vi "solar_type Set Items (Variants).vi"(4 "Include Cluster Prefix? (F)":bool, 6 "Prefix":string, 8 "error in (no error)":errorcluster, 9 "Keep Attributes? (F)":bool, 10 "Items":T1[](array[typedef]), 11 "Variant in":variant) -> (0 "error out":errorcluster, 3 "Variant out":variant)   [LabVIEW 2018]
doc: "This sets the Items into the Variant data."
uses:
  solar_type Item Type.ctl
  solar_type Item.ctl
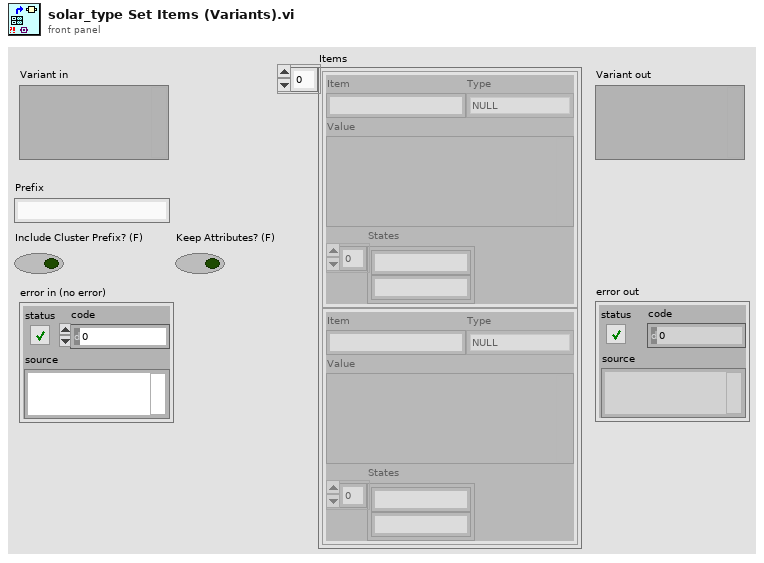
[diagram p1: front panel]
types:
  T1 = typedef "solar_type Item.ctl" = cluster{"Item":string, "Type":T2, "Value":variant, "States":string[]}
  T2 = typedef "solar_type Item Type.ctl" = enum16{"NULL", "UNKNOWN", "CLUSTER", "I8", "I16", "I32", "I64", "U8", "U16", "U32", "U64", "U8_ENUM", "U16_ENUM", "U32_ENUM", "SGL", "DBL", "BOOLEAN", "STRING", "PATH", "VISA", "TAG", "TIME", "I8_1D", "I16_1D", "I32_1D", "I64_1D", "U8_1D", "U16_1D", "U32_1D", "U64_1D", "U8_ENUM_1D", "U16_ENUM_1D", "U32_ENUM_1D", "SGL_1D", "DBL_1D", "BOOLEAN_1D", "STRING_1D", "PATH_1D", "VISA_1D", "TAG_1D", "TIME_1D", "I8_2D", "I16_2D", "I32_2D", "I64_2D", "U8_2D", "U16_2D", "U32_2D", "U64_2D", "U8_ENUM_2D", "U16_ENUM_2D", "U32_ENUM_2D", "SGL_2D", "DBL_2D", "BOOLEAN_2D", "STRING_2D", "PATH_2D", "VISA_2D", "TAG_2D", "TIME_2D"}
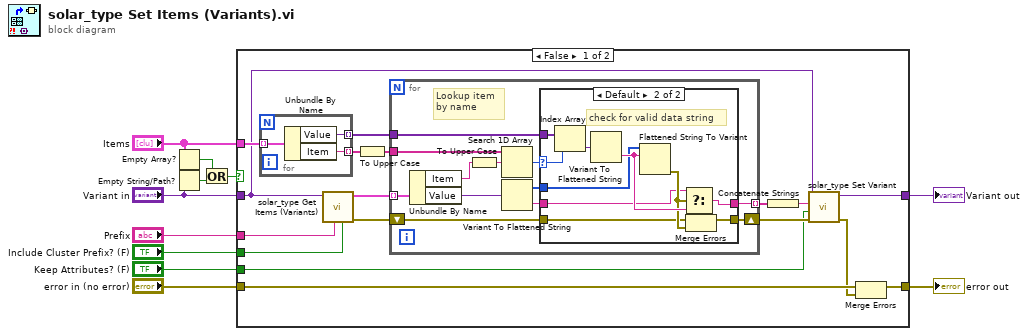
[diagram p0: block diagram]
diagram:
  n1 = Empty Array?(array="Items") -> (empty?=w1:bool)
  n2 = Empty String/Path?(string/path="Variant in") -> (empty?=w4:bool)
  n3 = Or(x=w1, y=w4) -> (x .or. y?=w3:bool)
  n4 = case shown="False" w3 {
    tunnel: "error in (no error)" -> [w27 w56]
    tunnel: [w26 w56] -> w10
    tunnel: "Prefix" -> [w25 _]
    tunnel: "Include Cluster Prefix? (F)" -> [w24 _]
    tunnel: "Items" -> [w21 _]
    tunnel: "Keep Attributes? (F)" -> [w15 _]
    tunnel: "Variant in" -> [w14 w57]
    tunnel: [w12 w57] -> w6
    frame False {
      n5 = for {
        tunnel: w21 -> [w55] mode=indexing
        tunnel: [w54] -> w28 mode=indexing
        tunnel: [w53] -> w16 mode=indexing
        n6 = Unbundle By Name(w55) -> ("Value"=w53:variant, "Item"=w54:string)
      }
      n7 = call "solar_type Get Items (Variants).vi"("Include Cluster Prefix? (F)"=w24, "Prefix"=w25, "Variant"=w14) -> ("error out"=w18:errorcluster, "Items"=w23:T1[])  [unwired: 5 in, 2 out]
      n8 = To Upper Case(1:w28) -> (0:w22:string[])
      n9 = for {
        tunnel: w23 -> [w39] mode=indexing
        tunnel: w22 -> [w37]
        tunnel: w16 -> [w36]
        tunnel: [w34] -> w20 mode=indexing
        shift-right: [w33] -> w17
        shift-left: w18 -> [w32]
        # "Lookup item\nby name"
        n10 = Unbundle By Name(w39) -> ("Item"=w40:string, "Value"=w31:variant)
        n11 = To Upper Case(1:w40) -> (0:w38:string)
        n12 = Search 1D Array(1D array=w37, element=w38) -> (index of element=w35:i32)  [unwired: 1 in]
        n13 = Variant To Flattened String(Variant=w31) -> (data string=w29:string, 1:w30:i16[])
        n14 = case shown="Default" w35 {
          selector: w35 -> [_ w51]
          tunnel: w36 -> [_ w52]
          tunnel: [w42 w49] -> w34
          tunnel: [w41 w47] -> w33
          tunnel: w32 -> [w41 w46]
          tunnel: w30 -> [_ w45]
          tunnel: w29 -> [w42 w44]
          frame -1 {
          }
          frame Default {
            # "check for valid data string"
            n15 = Index Array(array=w52, index=w51) -> (element=w43:variant)
            n16 = Variant To Flattened String(Variant=w43) -> (data string=w50:string)  [unwired: 1 out]
            n17 = Flattened String To Variant(6:w50, 7:w45) -> (0:w48:errorcluster)  [unwired: 1 in, 1 out]
            n18 = Select(t=w44, s=w48, f=w50) -> (s? t:f=w49:string)
            n19 = Merge Errors(w46, w48) -> (w47:errorcluster)
          }
        }
      }
      n20 = Concatenate Strings(w20) -> (w19:string)
      n21 = call "solar_type Set Variant.vi"("error in (no error)"=w17, "Keep Attributes? (F)"=w15, "Data String"=w19, "Variant in"=w14) -> ("error out"=w13:errorcluster, "Variant out"=w12:variant)  [unwired: 5 in, 1 out]
      n22 = Merge Errors(w27, w13) -> (w26:errorcluster)
    }
    frame True {
    }
  }
  "Variant out" <- w6
  "error out" <- w10
